vi "GameOption.vi"() -> ()   [LabVIEW 2017]
doc: "SubVI utilizada para mostrar um pop-up para o usuário de modo que ele possa escolher qual opção de jogo deseja - Player 1 x Player 2 ou Player 2 x Computador"
panel:
  in  "PxC":bool
  in  "PxP":bool
  # "Olá! Como você quer jogar?"
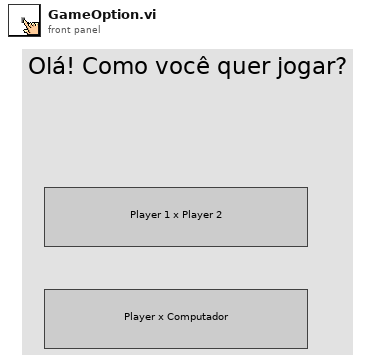
[diagram p1: front panel]
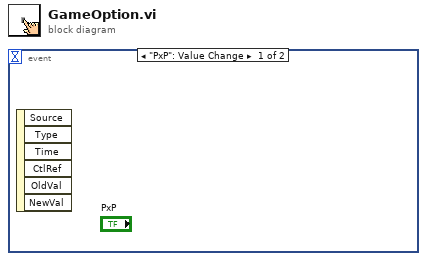
[diagram p0: block diagram]
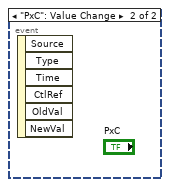
[diagram p2: hidden frame]
diagram:
  n1 = event shown="[0] \"PxP\": Value Change" {
    selector: _ -> [_ _]
    dyn-events: _ -> [_ _]
    timeout: _ -> [_ _]
    event "PxP": Value Change {
      n2 = event-data() -> ()  [unwired: 1 in, 6 out]
    }
    event "PxC": Value Change {
      n3 = event-data() -> ()  [unwired: 1 in, 6 out]
    }
  }
